vi "Send ADC.vi"(8 "error in (no error)":errorcluster, 9 "VISA resource name":refnum<visa-resource-name>, 10 "Channel ADC":u16, 11 "Cypress in":refnum<class "Cypress.lvclass">) -> (0 "error out":errorcluster, 1 "ADC Value":dbl, 2 "VISA resource name 2":refnum<visa-resource-name>, 3 "Cypress out":refnum<class "Cypress.lvclass">)   [LabVIEW 2020, in "Cypress.lvclass"]
uses:
  Cypress.lvclass
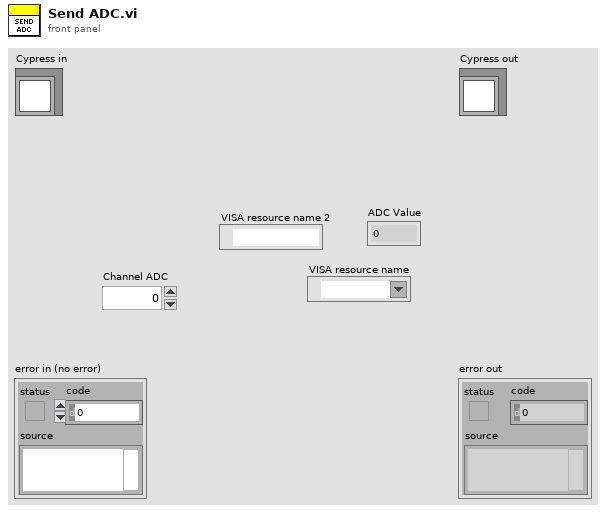
[diagram p1: front panel]
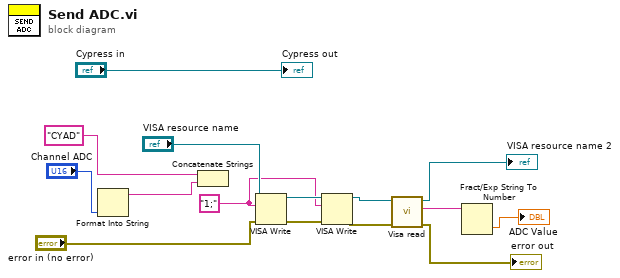
[diagram p0: block diagram]
diagram:
  w1 = "1;" ("write buffer")
  n1 = Format Into String("Channel ADC") -> (resulting string=w12:string)  [unwired: 3 in, 1 out]
  n2 = Concatenate Strings("CYAD", w12) -> ()  [unwired: 1 out]
  n3 = VISA Write(VISA resource name="VISA resource name", write buffer=w1, error in (no error)="error in (no error)") -> (VISA resource name out=w9:refnum<visa-resource-name>, error out=w11:errorcluster)  [unwired: 1 out]
  n4 = VISA Write(VISA resource name=w9, write buffer=w1, error in (no error)=w11) -> (VISA resource name out=w7:refnum<visa-resource-name>, error out=w6:errorcluster)  [unwired: 1 out]
  n5 = call "Visa read.vi"("error in (no error)"=w6, "VISA Refnum in"=w7) -> ("error out"=→"error out":errorcluster, "String"=w3:string, "VISA Refnum out"=→"VISA resource name 2":refnum<visa-resource-name>)  [unwired: 7 in]
  n6 = Fract/Exp String To Number(string=w3) -> (number=→"ADC Value":dbl)  [unwired: 3 in, 1 out]
  "Cypress out" <- "Cypress in"
